vi "ISA010State.vi"(8 "error in (no error)":errorcluster, 10 "state":string, 11 "Module ID":i32=-1) -> (0 "error out":errorcluster)   [LabVIEW 2017, in "ISA010_module.lvlib"]
doc: "_____\nCreated using Delacor QMH Event Scripter 3.1.0.29."
uses:
  ISA010_module.lvlib
  getISA010State Argument--cluster.ctl
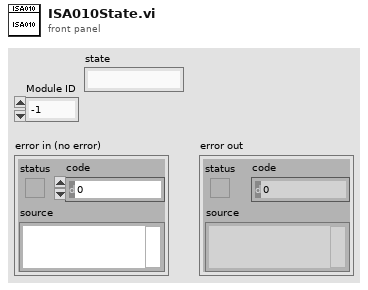
[diagram p1: front panel]
types:
  T1 = typedef "ISA010_module.lvlib/getISA010State Argument--cluster.ctl" = cluster{"Module ID":i32, "Boolean":bool, "state":string}
  T2 = typedef "ISA010_module.lvlib/Broadcast Events--cluster.ctl" = cluster{"Module Did Init":refnum<user-event>, "Status Updated":refnum<user-event>, "Error Reported":refnum<user-event>, "Module Did Stop":refnum<user-event>, "Update Module Execution Status":refnum<user-event>, "ISA010State":refnum<user-event>}
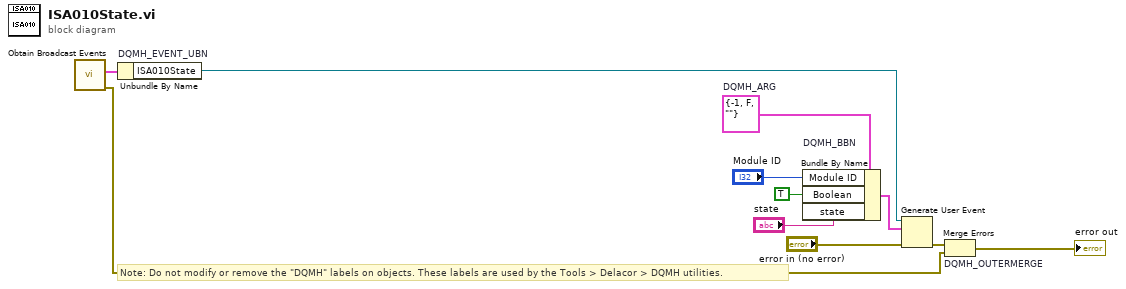
[diagram p0: block diagram]
diagram:
  w6 = T1 {"Module ID"=-1, "Boolean"=FALSE, "state"=""}  # DQMH_ARG
  # "Note: Do not modify or remove the \"DQMH\" labels on objects. These labels are used by the Tools > Delacor > DQMH utilities."
  n1 = call "Obtain Broadcast Events.vi"() -> ("error out"=w3:errorcluster, "ISA010_module Broadcast Events"=w2:T2)  [unwired: 10 in]
  n2 = Unbundle By Name "DQMH_EVENT_UBN"(w2) -> ("ISA010State"=w8:refnum<user-event>)
  n3 = Bundle By Name "DQMH_BBN"(cluster=w6, "Module ID"="Module ID", "Boolean"=TRUE, "state"="state") -> (w9:T1)
  n4 = Generate User Event(user event=w8, event data cluster=w9, error in="error in (no error)") -> (error out=w7:errorcluster)  [unwired: 1 in, 1 out]
  n5 = Merge Errors "DQMH_OUTERMERGE"(w7, w3) -> (→"error out":errorcluster)
